vi "RFmx_An_Harms_Disp.vi"(11 "Input_Spectrums":cluster{"x0":dbl, "dx":dbl, "y":sgl[]}[](array[cluster])) -> (3 "SFDR_Spectrum":cluster{"x0":dbl, "dx":dbl, "y":sgl[]}[](graph))   [LabVIEW 2014]
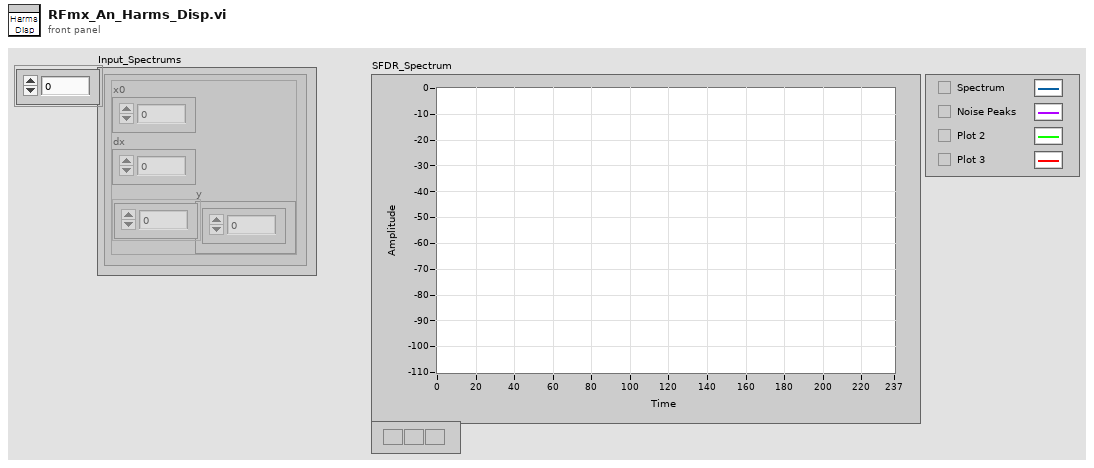
[diagram p1: front panel]
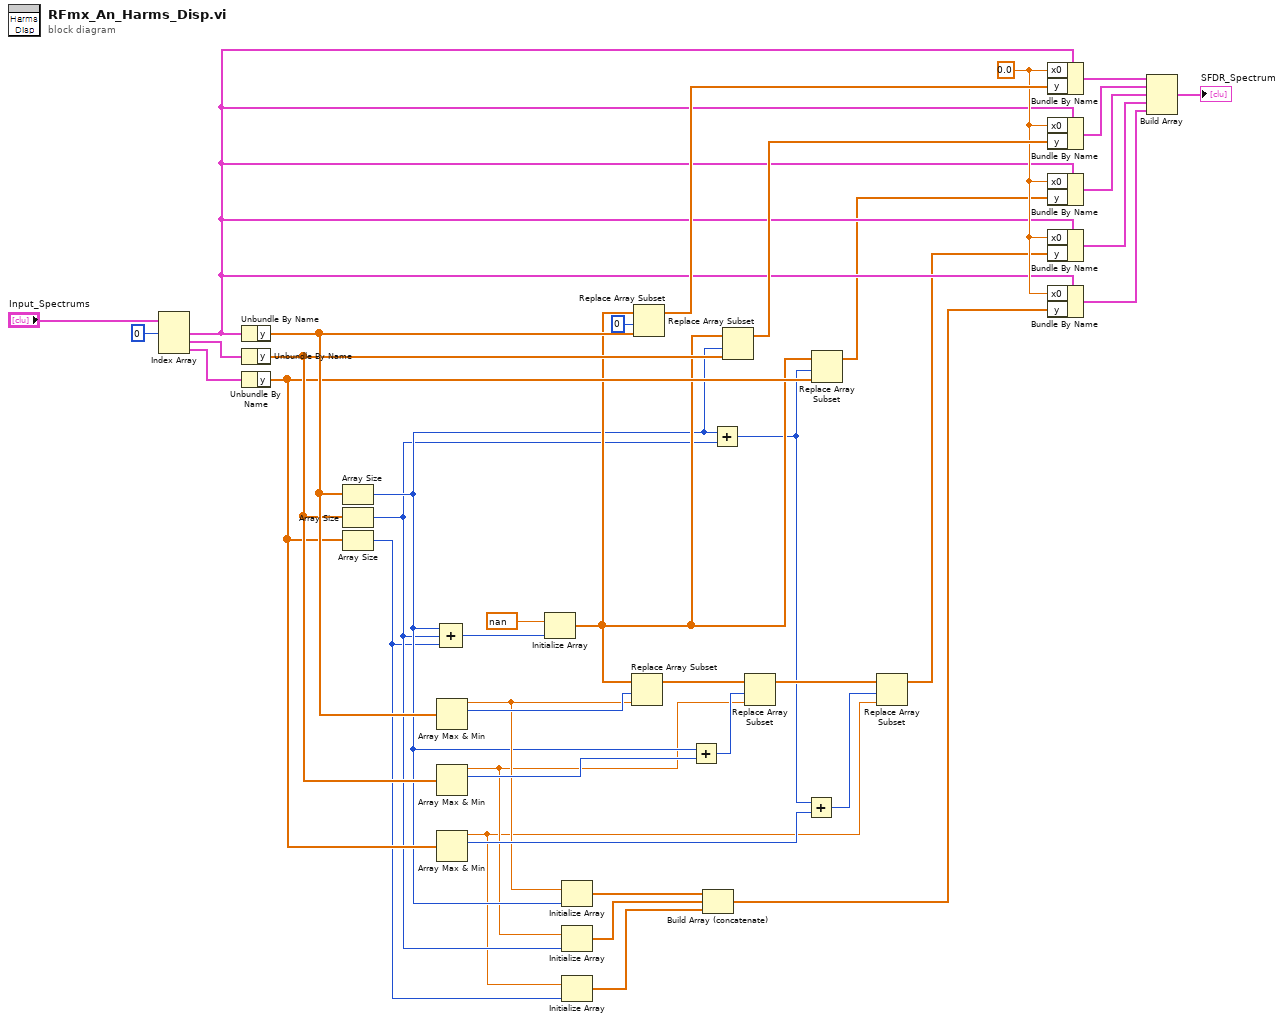
[diagram p0: block diagram]
diagram:
  w10 = 0.0 ("x0")
  n1 = Index Array(array="Input_Spectrums", index #1=0 ("index")) -> (element #1=w9:cluster{"x0":dbl, "dx":dbl, "y":sgl[]}, element #2=w39:cluster{"x0":dbl, "dx":dbl, "y":sgl[]}, element #3=w38:cluster{"x0":dbl, "dx":dbl, "y":sgl[]})  [unwired: 2 in]
  n2 = Unbundle By Name(w9) -> ("y"=w34:sgl[])
  n3 = Unbundle By Name(w39) -> ("y"=w33:sgl[])
  n4 = Unbundle By Name(w38) -> ("y"=w32:sgl[])
  n5 = Array Size(array=w34) -> (size(s)=w21:i32)
  n6 = Array Size(array=w33) -> (size(s)=w20:i32)
  n7 = Array Size(array=w32) -> (size(s)=w17:i32)
  n8 = Array Max & Min(array=w34) -> (max value=w22:sgl, max index (indices)=w30:i32)  [unwired: 2 out]
  n9 = Array Max & Min(array=w33) -> (max value=w19:sgl, max index (indices)=w27:i32)  [unwired: 2 out]
  n10 = Array Max & Min(array=w32) -> (max value=w18:sgl, max index (indices)=w24:i32)  [unwired: 2 out]
  n11 = Compound Arithmetic op=ADD(w21, w20, w17) -> (w37:i32)
  n12 = Initialize Array(sgl nan, w37) -> (w31:sgl[])
  n13 = Initialize Array(w22, w21) -> (w16:sgl[])
  n14 = Initialize Array(w19, w20) -> (w15:sgl[])
  n15 = Initialize Array(w18, w17) -> (w14:sgl[])
  n16 = Replace Array Subset(array=w31, new element=w22, index=w30) -> (w29:sgl[])
  n17 = Replace Array Subset(array=w31, new element=w34, index=0) -> (w13:sgl[])
  n18 = Add(x=w21, y=w27) -> (x+y=w26:i32)
  n19 = Build Array (concatenate)(w16, w15, w14) -> (w6:sgl[])
  n20 = Add(x=w21, y=w20) -> (x+y=w25:i32)
  n21 = Replace Array Subset(array=w31, new element=w33, index=w21) -> (w12:sgl[])
  n22 = Replace Array Subset(array=w29, new element=w19, index=w26) -> (w28:sgl[])
  n23 = Add(x=w25, y=w24) -> (x+y=w23:i32)
  n24 = Replace Array Subset(array=w31, new element=w32, index=w25) -> (w8:sgl[])
  n25 = Replace Array Subset(array=w28, new element=w18, index=w23) -> (w7:sgl[])
  n26 = Bundle By Name(cluster=w9, "x0"=w10, "y"=w13) -> (w11:cluster{"x0":dbl, "dx":dbl, "y":sgl[]})
  n27 = Bundle By Name(cluster=w9, "x0"=w10, "y"=w12) -> (w5:cluster{"x0":dbl, "dx":dbl, "y":sgl[]})
  n28 = Bundle By Name(cluster=w9, "x0"=w10, "y"=w8) -> (w4:cluster{"x0":dbl, "dx":dbl, "y":sgl[]})
  n29 = Bundle By Name(cluster=w9, "x0"=w10, "y"=w7) -> (w3:cluster{"x0":dbl, "dx":dbl, "y":sgl[]})
  n30 = Bundle By Name(cluster=w9, "x0"=w10, "y"=w6) -> (w2:cluster{"x0":dbl, "dx":dbl, "y":sgl[]})
  n31 = Build Array(w11, w5, w4, w3, w2) -> (→"SFDR_Spectrum":cluster{"x0":dbl, "dx":dbl, "y":sgl[]}[])
